vi "ExperimentMatlabEventHandlers.vi"(0 "Event Registration Refnum in":refnum<event-registration>, 1 "Controls[]":refnum<vi>[](array[refnum]), 3 "MEditor":refnum<k24>, 4 "ScriptFile":refnum<vi>, 5 "user event in":refnum<user-event>) -> ()   [LabVIEW 2017]
uses:
  C:/Code/CMCryoSysCode/CSharp/MatlabEditor/MatlabEditor/bin/Debug/MatlabEditor.dll
  CSharp/MatlabEditor/MatlabEditor/bin/Debug/MatlabEditor.dll
panel:
  in  "ExperimentID":string
  in  "Milliseconds \nTo Wait For \nEvents":i32=50
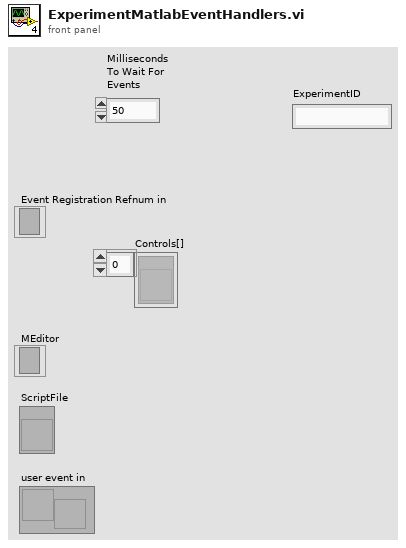
[diagram p1: front panel]
types:
  T1 = typedef "MatlabDataType.ctl" = enum16{"NotAMatlabType", "Real", "Complex", "String", "Boolean"}
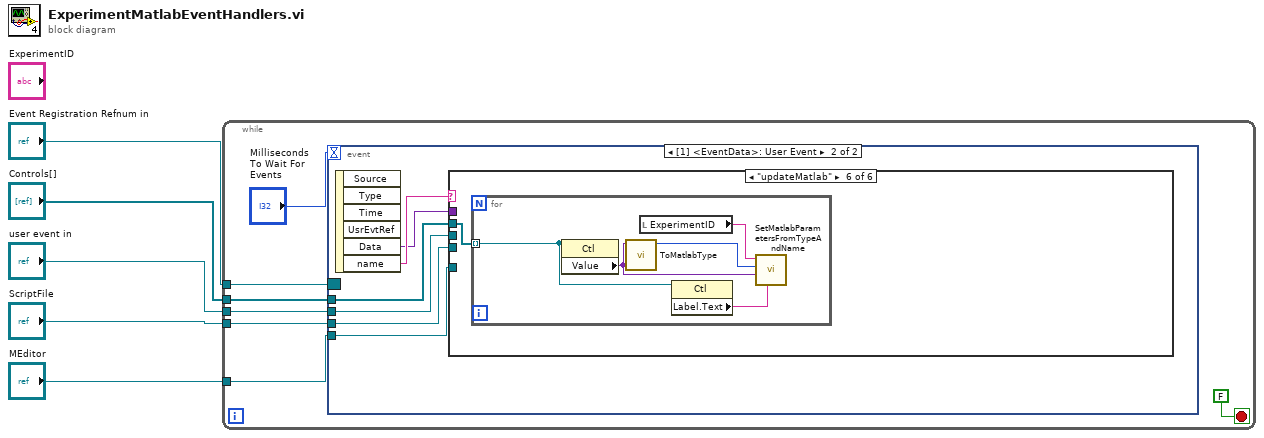
[diagram p0: block diagram]
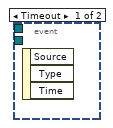
[diagram p2: hidden frame]
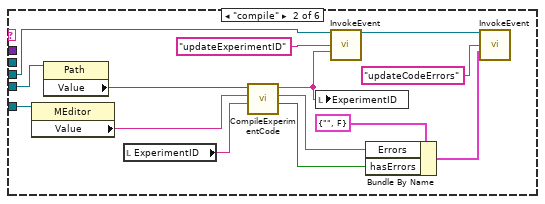
[diagram p4: hidden frame]
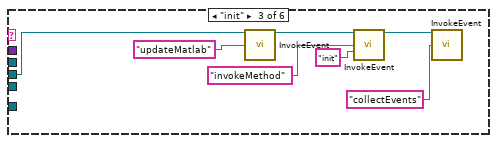
[diagram p5: hidden frame]
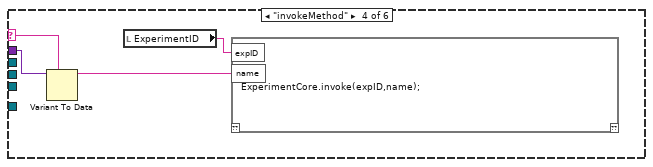
[diagram p6: hidden frame]
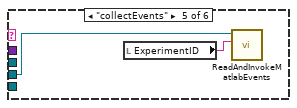
[diagram p7: hidden frame]
diagram:
  n1 = while {
    tunnel: "Event Registration Refnum in" -> [w11]
    tunnel: "user event in" -> [w10]
    tunnel: "MEditor" -> [w9]
    tunnel: "ScriptFile" -> [w8]
    tunnel: "Controls[]" -> [w6]
    stop <- FALSE stop-if-true
    n2 = event shown="[1] <EventData>: User Event" {
      selector: w11 -> [_ _]
      dyn-events: _ -> [_ _]
      timeout: "Milliseconds \nTo Wait For \nEvents" -> [_ _]
      tunnel: w10 -> [_ w16]
      tunnel: w9 -> [_ w15]
      tunnel: w8 -> [_ w14]
      tunnel: w6 -> [_ w13]
      event Timeout {
        n3 = event-data() -> ()  [unwired: 1 in, 3 out]
      }
      event User Event {
        n4 = event-data() -> ("Data"=w17:variant, "name"=w18:string)  [unwired: 1 in, 4 out]
        n5 = case shown="\"updateMatlab\"" w18 {
          selector: w18 -> [_ _ _ w42 _ _]
          tunnel: w16 -> [_ w25 w38 _ w45 _]
          tunnel: w17 -> [_ _ _ w43 _ _]
          tunnel: w15 -> [_ w20 _ _ _ _]
          tunnel: w14 -> [_ w32 _ _ _ _]
          tunnel: w13 -> [_ _ _ _ _ w46]
          frame "False", Default {
          }
          frame "compile" {
            n6 = property class="MEditor"(reference=w20) -> ("Value"=w21:string)  [unwired: 1 in, 2 out]
            n7 = property class="Path"(reference=w32) -> ("Value"=w31:path)  [unwired: 1 in, 2 out]
            n8 = local read "ExperimentID"() -> (w26:string)
            n9 = call "CompileExperimentCode.vi"("ExperimentID"=w26, "Value"=w21, "ScriptFile"=w31) -> ("Compiled?"=w29:bool, "Errors Text"=w22:string, "ExperimentID"=w19:string)  [unwired: 6 in]
            n10 = local write "ExperimentID"(w19) -> ()
            n11 = call "InvokeEvent.vi"("Event Stream In"=w25, "name"="updateExperimentID", "Data"=w19) -> ("Event Stream Out"=w24:refnum<user-event>)  [unwired: 11 in, 1 out]
            n12 = Bundle By Name(cluster=cluster{"Errors":string, "hasErrors":bool} {"Errors"="", "hasErrors"=FALSE}, "Errors"=w22, "hasErrors"=w29) -> (w27:cluster{"Errors":string, "hasErrors":bool})
            n13 = call "InvokeEvent.vi"("Event Stream In"=w24, "name"="updateCodeErrors", "Data"=w27) -> ()  [unwired: 11 in, 2 out]
          }
          frame "init" {
            n14 = call "InvokeEvent.vi"("Event Stream In"=w38, "name"="updateMatlab") -> ("Event Stream Out"=w37:refnum<user-event>)  [unwired: 12 in, 1 out]
            n15 = call "InvokeEvent.vi"("Event Stream In"=w37, "name"="invokeMethod", "Data"="init") -> ("Event Stream Out"=w34:refnum<user-event>)  [unwired: 11 in, 1 out]
            n16 = call "InvokeEvent.vi"("Event Stream In"=w34, "name"="collectEvents") -> ()  [unwired: 12 in, 2 out]
          }
          frame "invokeMethod" {
            n17 = Variant To Data(type=w42, Variant=w43) -> (data=w41:string)  [unwired: 1 in, 1 out]
            n18 = local read "ExperimentID"() -> (w40:string)
            n19 = script code="ExperimentCore.invoke(expID,name);"("expID"=w40, "name"=w41) -> ()  [unwired: 1 in, 1 out]
          }
          frame "collectEvents" {
            n20 = local read "ExperimentID"() -> (w44:string)
            n21 = call "ReadAndInvokeMatlabEvents.vi"("ExperimentID"=w44, "User Event in"=w45) -> ()  [unwired: 10 in]
          }
          frame "updateMatlab" {
            n22 = for {
              tunnel: w46 -> [w48] mode=indexing
              n23 = property class="Ctl"(reference=w48) -> ("Value"=w51:variant)  [unwired: 1 in, 2 out]
              n24 = call "ToMatlabType.vi"("Value"=w51) -> ("MatlabType"=w49:T1)  [unwired: 7 in, 3 out]
              n25 = local read "ExperimentID"() -> (w47:string)
              n26 = property class="Ctl"(reference=w48) -> ("Label.Text"=w50:string)  [unwired: 1 in, 2 out]
              n27 = call "SetMatlabParametersFromTypeAndName.vi"("Label.Text"=w50, "Value"=w51, "MatlabType"=w49, "ExperimentID"=w47) -> ()  [unwired: 8 in]
            }
          }
        }
      }
    }
  }
